vi "数组指定替换.vi"() -> ()   [LabVIEW 2018]
panel:
  out "字符串 2":string
  out "行":i32
  out "列":i32
  out "最小值":dbl
  out "最大值":dbl
  out "数组":i32[][](array[numeric])
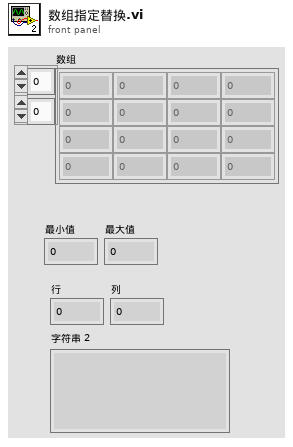
[diagram p1: front panel]
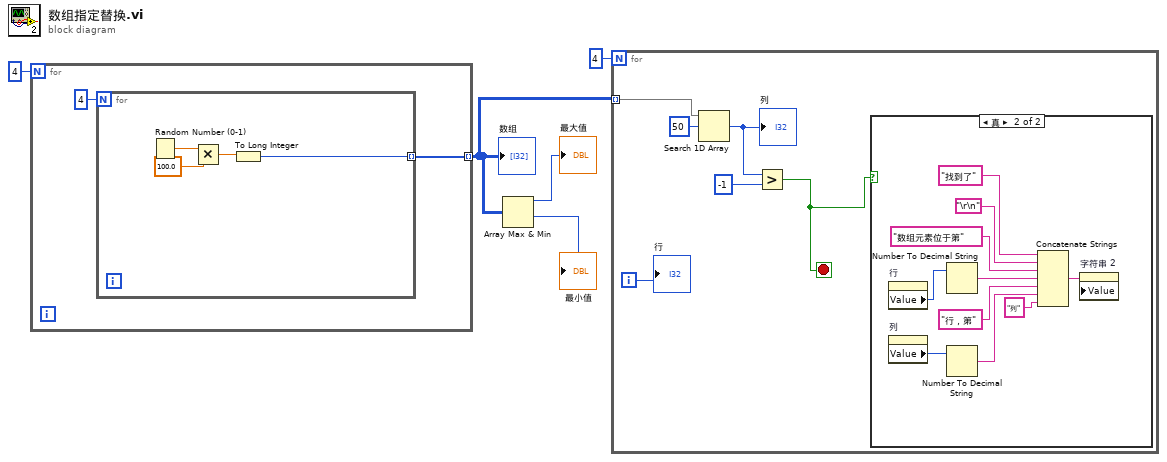
[diagram p0: block diagram]
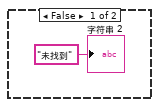
[diagram p2: hidden frame]
diagram:
  n1 = for {
    N: 4 -> [_]
    tunnel: [w6] -> w2 mode=indexing
    n2 = for {
      N: 4 -> [_]
      tunnel: [w8] -> w6 mode=indexing
      n3 = Random Number (0-1)() -> (number: 0 to 1=w11:dbl)
      n4 = Multiply(x=w11, y=100.0) -> (x*y=w9:dbl)
      n5 = To Long Integer(number=w9) -> (32bit integer=w8:i32)
    }
  }
  "数组" <- w2
  n6 = Array Max & Min(array=w2) -> (max value=→"最大值":i32, min value=→"最小值":i32)  [unwired: 2 out]
  n7 = for {
    N: 4 -> [_]
    tunnel: w2 -> [w17] mode=indexing
    i -> [w13]
    stop <- w12 stop-if-true
    n8 = Search 1D Array(1D array=w17, element=50 ("元素")) -> (index of element=w15:i32)  [unwired: 1 in]
    "列" <- w15
    n9 = Greater?(x=w15, y=-1) -> (0:w12:bool)
    n10 = case shown="真" w12 {
      frame False {
        "字符串 2" <- "未找到" ("字符串 2")
      }
      frame True {
        n11 = property on="行" class="DigNum (严格)"() -> ("Value"=w24:i32)  [unwired: 2 in, 2 out]
        n12 = property on="列" class="DigNum (严格)"() -> ("Value"=w22:i32)  [unwired: 2 in, 2 out]
        n13 = Number To Decimal String(number=w24) -> (decimal integer string=w23:string)  [unwired: 1 in]
        n14 = Number To Decimal String(number=w22) -> (decimal integer string=w20:string)  [unwired: 1 in]
        n15 = Concatenate Strings("找到了", "\r\n", "数组元素位于第", w23, "行，第", w20, "列") -> (w28:string)
        n16 = property on="字符串 2" class="Str"("Value"=w28) -> ()  [unwired: 2 in, 2 out]
      }
    }
    "行" <- w13
  }
